vi "Directional Speed Sensor.vi"() -> ()   [LabVIEW 2016]
doc: "This example demonstrates how to acquire a continuous amount of digital data based off of a sample clock.\n\nSome hardware (e.g. M Series DAQ) must use an external sample clock for digital tasks. To view a complete list of available sample clock sources, consult the Device Routes table in Measurement and Automation Explorer.\n\nFor instructions on how to connect your signals to the DAQ device, refer to your device documentation."
uses:
  <vilib>/Utility/error.llb/DialogType.ctl
  <vilib>/DAQmx/read.llb/DAQmx Read (Digital Wfm 1Chan NSamp).vi
  <vilib>/DAQmx/create/channels.llb/DAQmx Create Channel (DI-Digital Input).vi
  <vilib>/DAQmx/configure/timing.llb/DAQmx Timing (Sample Clock).vi
  <vilib>/DAQmx/miscellaneous.llb/DAQmx Fill In Error Info.vi
  <vilib>/Waveform/DWDTOps.llb/DWDT Digital to Analog.vi
panel:
  in  "Sampling rate":dbl=1000000.0
  out "Pass?":bool=TRUE
  in  "Backward pulse width(uS)":dbl=90.0
  in  "Forward pulse width(uS)":dbl=45.0
  out "number of high value samples in each pulse":i32[](array[numeric])=[46, 46, 46, 46, 46, 46, 46, 46, 46, 46, 46, 46, 46, 46, 46, 46, 46, 46, 46, 46, 46, 46, 46, 46, 46, 46, 46, 46, 46, 46, 46, 46, 46, 46, 46, 47, 46, 46, 46, 46, 46, 46, 46, 46, 46, 46, 46, 46, 46, 46, 46, 46, 46, 46, 46, 46, 46, 46]
  out "Waveform Graph":waveform(dbl)(graph)={"t0"=timestamp(3585136994.4907956 s since 1904-01-01), "dt"=9.9999999999997e-07, "Y"=array[1000000 elements], "attributes"=variant("NI_ChannelName"=variant(string "cDAQ1Mod1/port0/line2"), "NI_LineNames"=variant(string "cDAQ1Mod1/port0/line2"))}
  out "indices of samples equal to 0":i32[](array[numeric])
  in  "Duration":i32=1
  in  "RPM":dbl=120.0
  in  "Sample Clock Source":tag="OnboardClock"
  in  "Line(s)":tag="cDAQ1Mod1/port0/line2"
  # "This test checks if pulse width is consisstent within tolerance with different RPMs"
  # "Channel Settings"
  # "Acquired Data"
  # "Timing Settings"
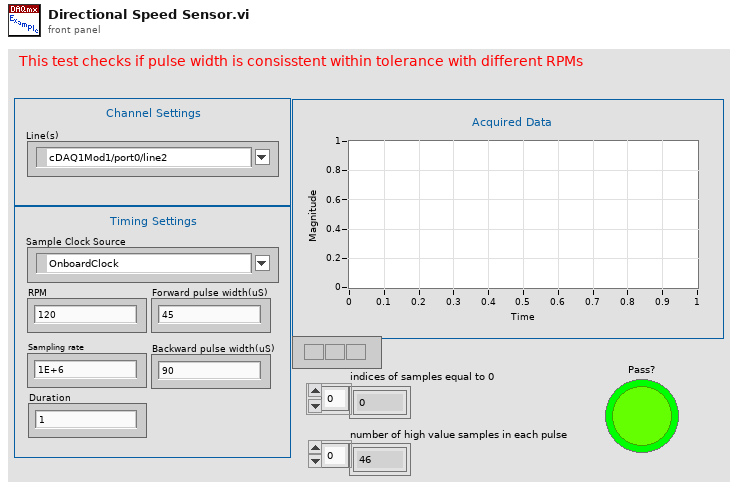
[diagram p1: front panel]
types:
  T1 = typedef "DialogType.ctl" = u16
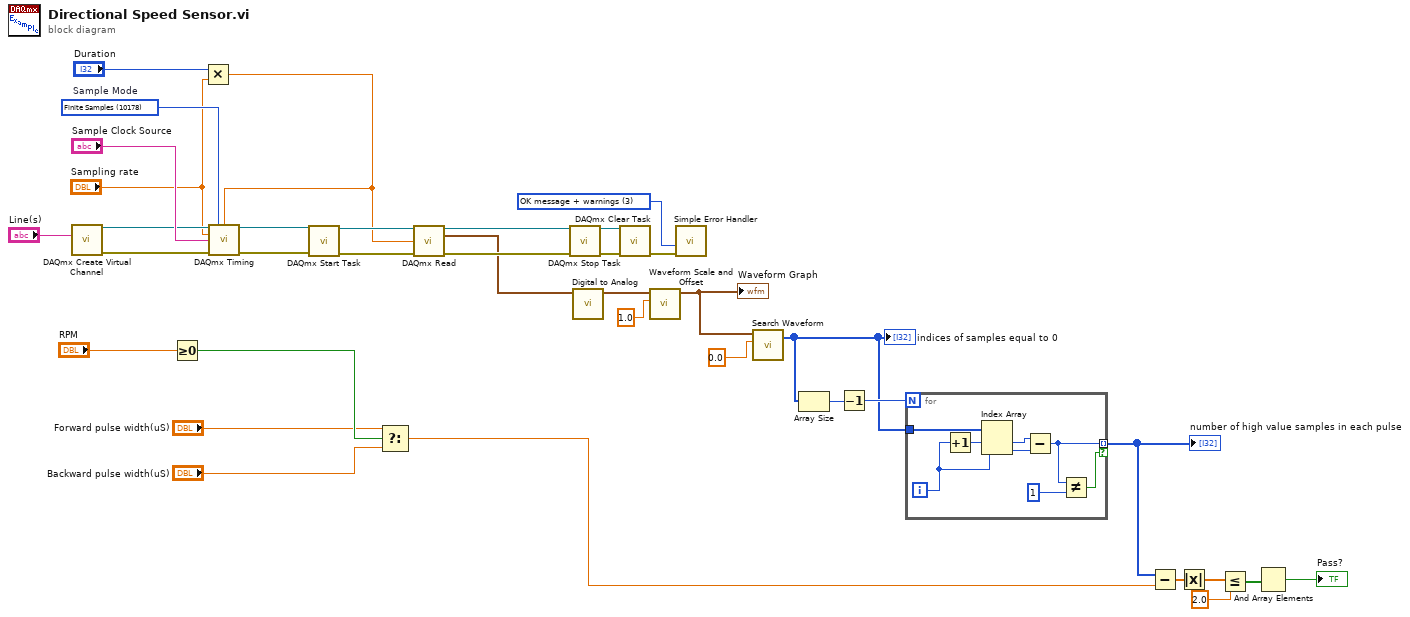
[diagram p0: block diagram]
diagram:
  w25 = T1 3 items=["no dialog", "OK message", "continue or stop message", "OK message + warnings", "continue/stop + warnings"] ("type of dialog (OK msg:1)")
  w35 = 10178 items=["Finite Samples"=10178, "Continuous Samples"=10123, "Hardware Timed Single Point"=12522]  # Sample Mode
  n1 = call-poly <vilib>:"DAQmx Create Virtual Channel.vi"("lines"="Line(s)") -> ("task out"=w33:refnum<k21>, "error out"=w32:errorcluster)  [unwired: 13 in]
  n2 = Greater Or Equal To 0?(x="RPM") -> (x >= 0?=w12:bool)
  n3 = Multiply(x="Duration", y="Sampling rate") -> (x*y=w15:dbl)
  n4 = call-poly <vilib>:"DAQmx Timing.vi"("task/channels in"=w33, "sample mode"=w35, "samples per channel"=w15, "rate"="Sampling rate", "source"="Sample Clock Source", "error in"=w32) -> ("task out"=w24:refnum<k21>, "error out"=w23:errorcluster)  [unwired: 8 in]
  n5 = call <vilib>:"DAQmx Start Task.vi"("task/channels in"=w24, "error in"=w23) -> ("task out"=w30:refnum<k21>, "error out"=w31:errorcluster)  [unwired: 12 in]
  n6 = Select(t="Forward pulse width(uS)", s=w12, f="Backward pulse width(uS)") -> (s? t:f=w2:dbl)
  n7 = call-poly <vilib>:"DAQmx Read.vi"("task/channels in"=w30, "number of samples per channel"=w15, "error in"=w31) -> ("task out"=w27:refnum<k21>, "data"=w16:digitalwaveform, "error out"=w26:errorcluster)  [unwired: 10 in]
  n8 = call <vilib>:"DAQmx Stop Task.vi"("task/channels in"=w27, "error in"=w26) -> ("task out"=w29:refnum<k21>, "error out"=w28:errorcluster)  [unwired: 12 in]
  n9 = call-poly <vilib>:"Digital to Analog.vi"("digital waveform"=w16) -> ("analog waveform"=w22:waveform(dbl))  [unwired: 7 in, 3 out]
  n10 = call <vilib>:"DAQmx Clear Task.vi"("task in"=w29, "error in"=w28) -> ("error out"=w37:errorcluster)  [unwired: 13 in]
  n11 = call <vilib>:"Waveform Scale and Offset.vi"("offset"=1.0, "waveform in"=w22) -> ("waveform out"=w14:waveform(dbl))  [unwired: 8 in, 1 out]
  "Waveform Graph" <- w14
  n12 = call <vilib>:"Simple Error Handler.vi"("type of dialog (OK msg:1)"=w25, "error in (no error)"=w37) -> ()  [unwired: 3 in, 5 out]
  n13 = call <vilib>:"Search Waveform.vi"("value"=0.0, "waveform in"=w14) -> ("indices of fits"=w18:i32[])  [unwired: 4 in, 5 out]
  "indices of samples equal to 0" <- w18
  n14 = Array Size(array=w18) -> (size(s)=w17:i32)
  n15 = Decrement(x=w17) -> (x-1=w19:i32)
  n16 = for {
    N: w19 -> [_]
    tunnel: w18 -> [w45]
    tunnel: [w38] -> w6 mode=indexing if=w39
    i -> [w40]
    n17 = Increment(x=w40) -> (x+1=w44:i32)
    n18 = Index Array(array=w45, index #1=w44, index #2=w40) -> (element #1=w42:i32, element #2=w43:i32)
    n19 = Subtract(x=w42, y=w43) -> (x-y=w38:i32)
    n20 = Not Equal?(x=w38, y=1) -> (x != y?=w39:bool)
  }
  "number of high value samples in each pulse" <- w6
  n21 = Subtract(x=w6, y=w2) -> (x-y=w7:dbl[])
  n22 = Absolute Value(x=w7) -> (abs(x)=w8:dbl[])
  n23 = Less Or Equal?(x=w8, y=2.0) -> (x <= y?=w5:bool[])
  n24 = And Array Elements(Boolean array=w5) -> (logical AND=→"Pass?":bool)
